vi "Set Impulse Plane.vi"(10 "Impulse Plane":T1, 11 "Reference in":T2) -> (3 "Reference out":T2)   [LabVIEW 2016, in "Impulse Data.lvclass"]
uses:
  Impulse Data.lvclass
  Instance handle.ctl
  type-defs/TD_Impulse Planes.ctl
  Impulse Data.lvclass/Impulse Data.ctl
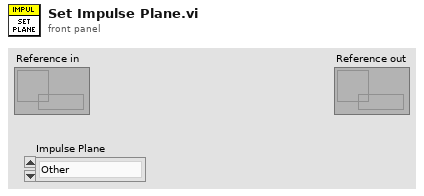
[diagram p1: front panel]
types:
  T1 = typedef "TD_Impulse Planes.ctl" = enum16{"Other", "Yaw", "Pitch", "Roll", "LARP", "RALP"}
  T2 = typedef "Impulse Data.lvclass/Instance handle.ctl" = refnum<data-value>
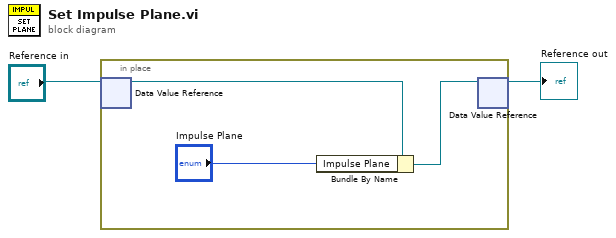
[diagram p0: block diagram]
diagram:
  n1 = in-place {
    n2 = in-place-dvr #1("Reference in") -> (w5:refnum<class "Impulse Data.lvclass">)  [unwired: 1 out]
    n3 = Bundle By Name(cluster=w5, "Impulse Plane"="Impulse Plane") -> (w4:refnum<class "Impulse Data.lvclass">)
    n4 = in-place-dvr #1(w4) -> (→"Reference out":T2)  [unwired: 1 out]
  }
